vi "image_acq.vi"() -> ()   [LabVIEW 2011]
uses:
  <vilib>/userdefined/High Color/IMAQdx.ctl
  <vilib>/vision/driver/NI_Vision_Acquisition_Software.lvlib
panel:
  out "Session Out":T1
  out "error out":errorcluster
  in  "error in":errorcluster
  in  "Session In":T1
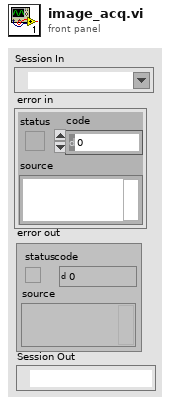
[diagram p1: front panel]
types:
  T1 = typedef "IMAQdx.ctl" = refnum<k21>
  T2 = typedef "IMAQ Image.ctl" = refnum<image>
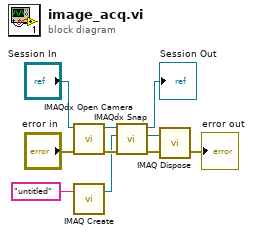
[diagram p0: block diagram]
diagram:
  n1 = call <vilib>:"IMAQdx Open Camera.vi"("error in"="error in", "Session In"="Session In") -> ("error out"=w7:errorcluster, "Session Out"=w8:T1)  [unwired: 8 in]
  n2 = call "IMAQ Create"("Image Name"="untitled") -> ("New Image"=w6:T2)  [unwired: 4 in, 1 out]
  n3 = call <vilib>:"IMAQdx Snap.vi"("error in"=w7, "Image In"=w6, "Session In"=w8) -> ("error out"=w3:errorcluster, "Image Out"=w4:T2, "Session Out"=→"Session Out":T1)  [unwired: 6 in]
  n4 = call "IMAQ Dispose"("Image"=w4, "error in (no error)"=w3) -> ("error out"=→"error out":errorcluster)  [unwired: 4 in]
